vi "CRYCalc minimum.vi"(6 "Work in":u16, 7 "Step Setup VI No":i32, 8 "Statistic Run Number":i32, 11 "Data in":T1 {"Z data" items=["dB", "Lin"]; "X data" items=["dB", "Lin"]; "Y data" items=["dB", "Lin"]; "Z dB ref" format="%.1f"; "Z axis" items=["Log", "Lin"]; "X dB ref" format="%.1f"; "X axis" items=["Log", "Lin"]; "Y axis" items=["Log", "Lin"]; "Y dB ref" format="%.1f"; "Curve"."z" format="%.2f"; "Curve"."y" format="%.2f"; "Curve"."x" format="%.2f"}) -> (3 "Minimum Out":T1 {"Z data" items=["dB", "Lin"]; "X data" items=["dB", "Lin"]; "Y data" items=["dB", "Lin"]; "Z dB ref" format="%.1f"; "Z axis" items=["Log", "Lin"]; "X dB ref" format="%.1f"; "X axis" items=["Log", "Lin"]; "Y axis" items=["Log", "Lin"]; "Y dB ref" format="%.1f"; "Curve"."z" format="%.2f"; "Curve"."y" format="%.2f"; "Curve"."x" format="%.2f"})   [LabVIEW 2013]
uses:
  Typedef Control/CRYData Cluster Array.ctl
  Typedef Control/CRYData Cluster.ctl
  CRYStatistics Global.vi
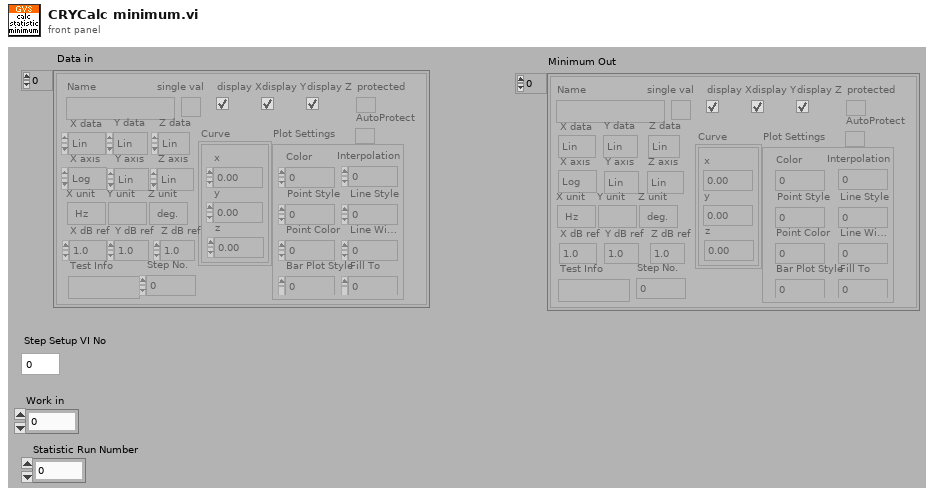
[diagram p1: front panel]
types:
  T1 = typedef "CRYData Cluster Array.ctl" = T2[]
  T2 = typedef "CRYData Cluster.ctl" = cluster{"Name":string, "Curve":cluster{"x":dbl, "y":dbl, "z":dbl}[], "X data":u16, "Y data":u16, "Z data":u16, "X axis":u16, "Y axis":u16, "Z axis":u16, "X unit":string, "Y unit":string, "Z unit":string, "X dB ref":dbl, "Y dB ref":dbl, "Z dB ref":dbl, "single val":bool, "protected":bool, "display X":bool, "display Y":bool, "display Z":bool, "Test Info":string, "Step No.":i32, "Plot Settings":cluster{"Color":u32, "Interpolation":u8, "Point Style":u8, "Line Style":u8, "Point Color":u32, "Line Width":u8, "Bar Plot Style":u8, "Fill To":i16}, "AutoProtect":bool}
  T3 = enum32{"English", "Chinese", "Korean", "Japanese", "Russian", "Chinese traditional"}
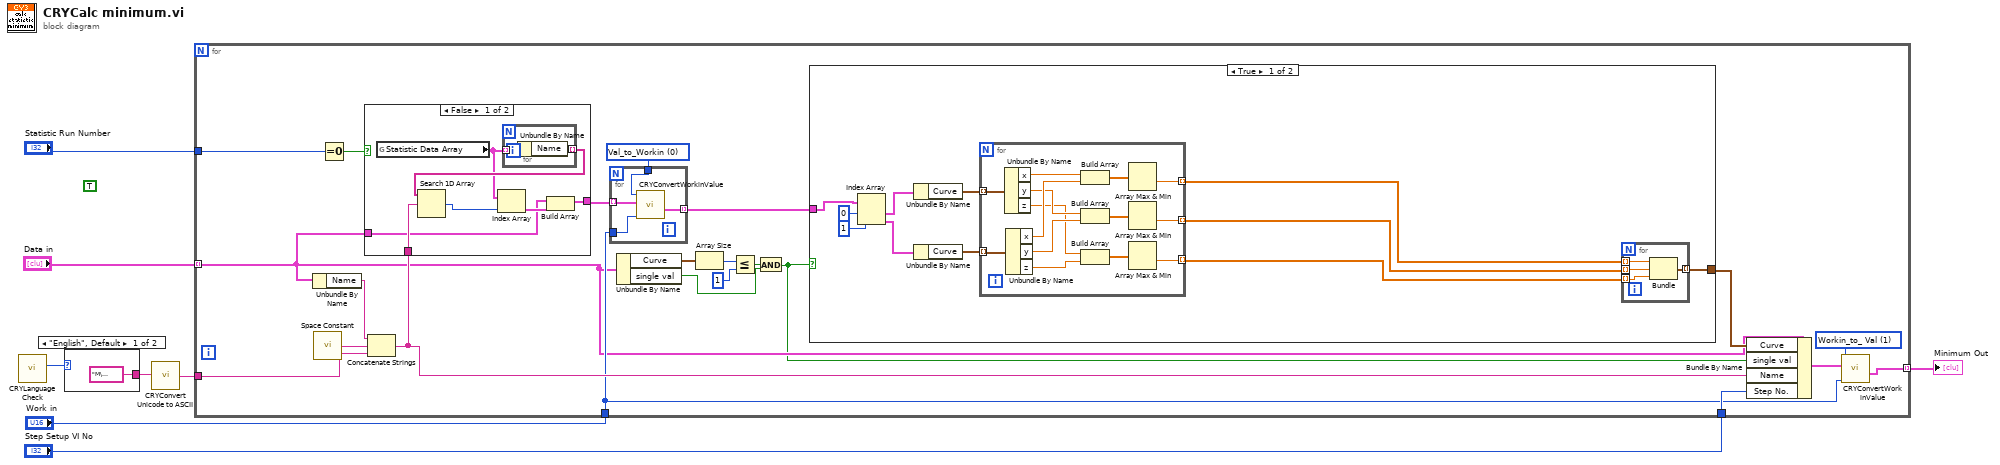
[diagram p0: block diagram]
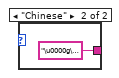
[diagram p2: hidden frame]
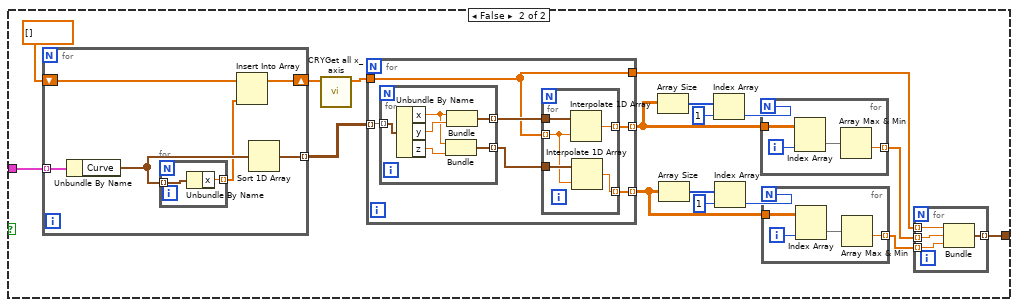
[diagram p3: hidden frame]
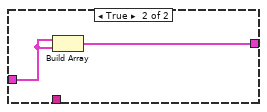
[diagram p4: hidden frame]
diagram:
  (unwired) TRUE
  n1 = call "CRYLanguage Check.vi"() -> ("Language"=w3:T3)  [unwired: 10 in, 1 out]
  n2 = case shown="\"English\", Default" w3 {
    tunnel: ["M\u0000i\u0000n\u0000" ("format string") "\u0000g\u000f\\<P" ("format string")] -> w4
    frame "English", Default {
    }
    frame "Chinese" {
    }
  }
  n3 = call "CRYConvert Unicode to ASCII.vi"("Unicode"=w4) -> ("ASCII"=w2:string)  [unwired: 4 in]
  n4 = for {
    tunnel: "Data in" -> [w12] mode=indexing
    tunnel: [w21] -> w8 mode=indexing
    tunnel: "Step Setup VI No" -> [w30]
    tunnel: "Statistic Run Number" -> [w29]
    tunnel: w2 -> [w25]
    tunnel: "Work in" -> [w18]
    w19 = u16 0 items=["Val_to_Workin", "Workin_to_ Val"] ("Type")
    w20 = u16 1 items=["Val_to_Workin", "Workin_to_ Val"] ("Type")
    n5 = Unbundle By Name(w12) -> ("Name"=w27:string)
    n6 = call <vilib>:"Space Constant.vi"() -> ("String"=w28:string)
    n7 = Equal To 0?(x=w29) -> (x = 0?=w26:bool)
    n8 = Concatenate Strings(w27, w28, w25) -> (w31:string)
    n9 = case shown="False" w26 {
      tunnel: w12 -> [w120 w130]
      tunnel: [w122 w129] -> w24
      tunnel: w31 -> [w126 _]
      frame False {
        n10 = global read "CRYStatistics Global.vi" "Statistic Data Array"() -> (w124:T1)
        n11 = for {
          tunnel: w124 -> [w128] mode=indexing
          tunnel: [w127] -> w125 mode=indexing
          n12 = Unbundle By Name(w128) -> ("Name"=w127:string)
        }
        n13 = Search 1D Array(1D array=w125, element=w126) -> (index of element=w123:i32)  [unwired: 1 in]
        n14 = Index Array(array=w124, index=w123) -> (element=w121:T2)
        n15 = Build Array(w120, w121) -> (w122:T2[])
      }
      frame True {
        n16 = Build Array(w130, w130) -> (w129:T2[])
      }
    }
    n17 = for {
      tunnel: w24 -> [w119] mode=indexing
      tunnel: [w118] -> w23 mode=indexing
      tunnel: w18 -> [w117]
      tunnel: w19 -> [w116]
      n18 = call "CRYConvertWorkinValue.vi"("Work in"=w117, "In"=w119, "Type"=w116) -> ("Out"=w118:T2)  [unwired: 8 in]
    }
    n19 = Unbundle By Name(w12) -> ("Curve"=w17:cluster{"x":dbl, "y":dbl, "z":dbl}[], "single val"=w13:bool)
    n20 = Array Size(array=w17) -> (size(s)=w16:i32)
    n21 = Less Or Equal?(x=w16, y=1) -> (x <= y?=w14:bool)
    n22 = And(x=w14, y=w13) -> (x .and. y?=w11:bool)
    n23 = case shown="True" w11 {
      tunnel: [w33 w69] -> w32
      tunnel: w23 -> [w34 w62]
      frame True {
        n24 = Index Array(array=w34, index #1=0 ("index"), index #2=1 ("index")) -> (element #1=w37:T2, element #2=w38:T2)
        n25 = Unbundle By Name(w37) -> ("Curve"=w39:cluster{"x":dbl, "y":dbl, "z":dbl}[])
        n26 = Unbundle By Name(w38) -> ("Curve"=w40:cluster{"x":dbl, "y":dbl, "z":dbl}[])
        n27 = for {
          tunnel: w39 -> [w57] mode=indexing
          tunnel: w40 -> [w56] mode=indexing
          tunnel: [w46] -> w41 mode=indexing
          tunnel: [w45] -> w42 mode=indexing
          tunnel: [w44] -> w43 mode=indexing
          n28 = Unbundle By Name(w57) -> ("x"=w55:dbl, "y"=w53:dbl, "z"=w51:dbl)
          n29 = Unbundle By Name(w56) -> ("x"=w54:dbl, "y"=w52:dbl, "z"=w50:dbl)
          n30 = Build Array(w55, w54) -> (w49:dbl[])
          n31 = Build Array(w53, w52) -> (w48:dbl[])
          n32 = Build Array(w51, w50) -> (w47:dbl[])
          n33 = Array Max & Min(array=w49) -> (min value=w46:dbl)  [unwired: 3 out]
          n34 = Array Max & Min(array=w48) -> (min value=w45:dbl)  [unwired: 3 out]
          n35 = Array Max & Min(array=w47) -> (min value=w44:dbl)  [unwired: 3 out]
        }
        n36 = for {
          tunnel: [w61] -> w33 mode=indexing
          tunnel: w41 -> [w60] mode=indexing
          tunnel: w42 -> [w59] mode=indexing
          tunnel: w43 -> [w58] mode=indexing
          n37 = Bundle(w60, w59, w58) -> (w61:cluster{dbl, dbl, dbl})  [unwired: 1 out]
        }
      }
      frame False {
        n38 = for {
          tunnel: [w91] -> w75 mode=indexing
          tunnel: w62 -> [w92] mode=indexing
          shift-right: [w94] -> w68
          shift-left: dbl[] [] ("x_Array") -> [w93]
          n39 = Unbundle By Name(w92) -> ("Curve"=w96:cluster{"x":dbl, "y":dbl, "z":dbl}[])
          n40 = for {
            tunnel: w96 -> [w97] mode=indexing
            tunnel: [w98] -> w95 mode=indexing
            n41 = Unbundle By Name(w97) -> ("x"=w98:dbl)
          }
          n42 = Insert Into Array(array=w93, new element=w95) -> (w94:dbl[])  [unwired: 1 in]
          n43 = Sort 1D Array(array=w96) -> (sorted array=w91:cluster{"x":dbl, "y":dbl, "z":dbl}[])
        }
        n44 = call "CRYGet all x_axis.vi"("x_Array in"=w68) -> ("X_axis out"=w74:dbl[])  [unwired: 1 in, 9 out]
        n45 = for {
          tunnel: w75 -> [w100] mode=indexing
          tunnel: [w104] -> w77 mode=indexing
          tunnel: w74 -> [w99]
          tunnel: [w99] -> w78
          tunnel: [w101] -> w64 mode=indexing
          n46 = for {
            tunnel: [w109] -> w103 mode=indexing
            tunnel: w100 -> [w108] mode=indexing
            tunnel: [w105] -> w102 mode=indexing
            n47 = Unbundle By Name(w108) -> ("x"=w106:dbl, "y"=w110:dbl, "z"=w107:dbl)
            n48 = Bundle("x"=w106, "z"=w107) -> (w105:cluster{"x":dbl, "z":dbl})  [unwired: 1 out]
            n49 = Bundle("x"=w106, "y"=w110) -> (w109:cluster{"x":dbl, "y":dbl})  [unwired: 1 out]
          }
          n50 = for {
            tunnel: [w115] -> w104 mode=indexing
            tunnel: w103 -> [w114]
            tunnel: w99 -> [w112] mode=indexing
            tunnel: w102 -> [w113]
            tunnel: [w111] -> w101 mode=indexing
            n51 = Interpolate 1D Array(1:w112, 2:w114) -> (0:w115:dbl)
            n52 = Interpolate 1D Array(1:w112, 2:w113) -> (0:w111:dbl)
          }
        }
        n53 = Array Size(array=w77) -> (size(s)=w73:i32[])
        n54 = Array Size(array=w64) -> (size(s)=w65:i32[])
        n55 = Index Array(array=w73, index=1) -> (element=w72:i32)
        n56 = Index Array(array=w65, index=1) -> (element=w66:i32)
        n57 = for {
          N: w72 -> [_]
          tunnel: w77 -> [w90]
          tunnel: [w87] -> w70 mode=indexing
          i -> [w88]
          n58 = Index Array(array=w90, index (col)=w88) -> (element=w89:dbl[])  [unwired: 1 in]
          n59 = Array Max & Min(array=w89) -> (min value=w87:dbl)  [unwired: 3 out]
        }
        n60 = for {
          N: w66 -> [_]
          tunnel: w64 -> [w82]
          tunnel: [w79] -> w63 mode=indexing
          i -> [w80]
          n61 = Index Array(array=w82, index (col)=w80) -> (element=w81:dbl[])  [unwired: 1 in]
          n62 = Array Max & Min(array=w81) -> (min value=w79:dbl)  [unwired: 3 out]
        }
        n63 = for {
          tunnel: w70 -> [w85] mode=indexing
          tunnel: [w86] -> w69 mode=indexing
          tunnel: w78 -> [w84] mode=indexing
          tunnel: w63 -> [w83] mode=indexing
          n64 = Bundle("x"=w84, w85, w83) -> (w86:cluster{"x":dbl, dbl, dbl})  [unwired: 1 out]
        }
      }
    }
    n65 = Bundle By Name(cluster=w12, "Curve"=w32, "single val"=w11, "Name"=w31, "Step No."=w30) -> (w22:T2)
    n66 = call "CRYConvertWorkinValue.vi"("Work in"=w18, "In"=w22, "Type"=w20) -> ("Out"=w21:T2)  [unwired: 8 in]
  }
  "Minimum Out" <- w8
